vi "LJM_eNames.vi"(0 "Handle In":i32, 1 "NumFrames":i32=-1, 5 "aNames":string[](array[string]), 9 "aValuesIn":dbl[](array[numeric]) format="%.2f", 11 "error in":errorcluster, 12 "aWrites":i32[](array[ring]) items=["Read", "Write"], 13 "aNumValues":i32[](array[numeric])) -> (4 "Handle Out":i32, 10 "aValuesOut":dbl[](array[numeric]) format="%.2f", 14 "ErrorAddress":i32, 15 "error out":errorcluster)   [LabVIEW 2020]
panel:
  # "This function does not check or modify the aValuesIn array.  You must initialize it properly.  We recommend\nalways using eNames2D in LabVIEW rather than eNames."
  # "1/20/2015:  Default value of NumFrames changed to -1.  If\nNumFrames = -1, then the NumFrames control is ignored\nand the size of aNames/aAddresses is used to determine how\nmany frames there are."
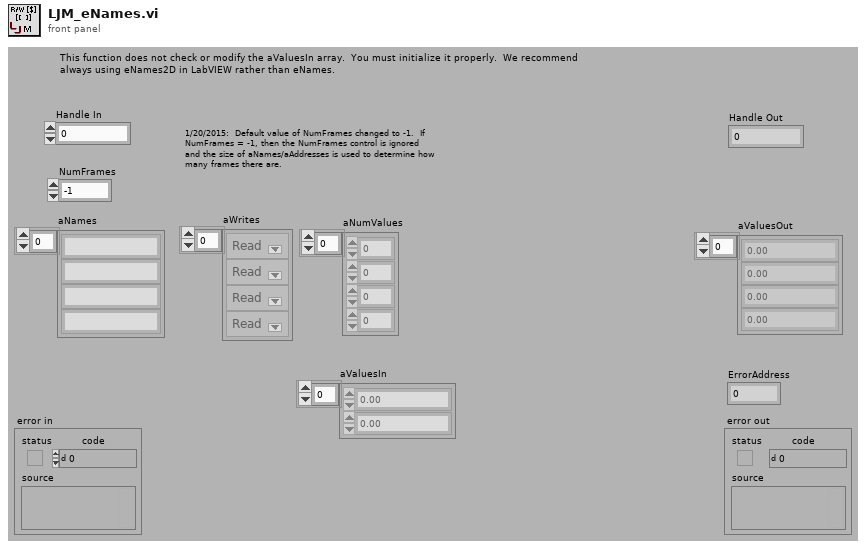
[diagram p1: front panel]
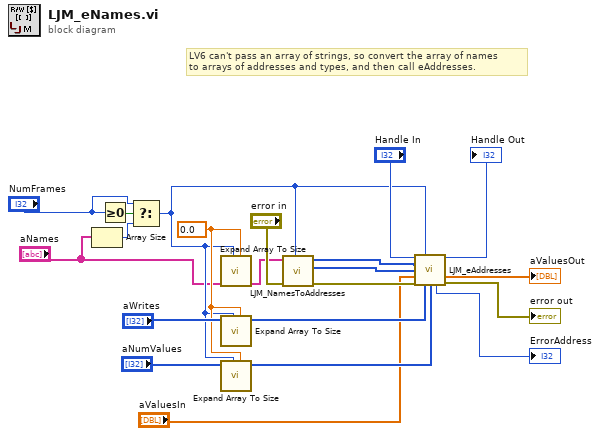
[diagram p0: block diagram]
diagram:
  w7 = 0.0 ("Default Value")
  # "LV6 can't pass an array of strings, so convert the array of names\nto arrays of addresses and types, and then call eAddresses."
  n1 = Array Size(array="aNames") -> (size(s)=w5:i32)
  n2 = Greater Or Equal To 0?(x="NumFrames") -> (x >= 0?=w4:bool)
  n3 = Select(t="NumFrames", s=w4, f=w5) -> (s? t:f=w3:i32)
  n4 = call "Expand Array To Size.vi"("Default Value"=w7, "# Elements"=w3, "String Array In"="aNames") -> ("String Array Out"=w18:string[])  [unwired: 4 in, 4 out]
  n5 = call "Expand Array To Size.vi"("Default Value"=w7, "# Elements"=w3, "I32 Array In"="aWrites") -> ("I32 Array Out"=w12:i32[])  [unwired: 4 in, 4 out]
  n6 = call "Expand Array To Size.vi"("Default Value"=w7, "# Elements"=w3, "I32 Array In"="aNumValues") -> ("I32 Array Out"=w11:i32[])  [unwired: 4 in, 4 out]
  n7 = call "LJM_NamesToAddresses.vi"("NumFrames (Auto-Detect)"=w3, "error in"="error in", "aNames"=w18) -> ("error out"=w17:errorcluster, "aTypes"=w13:i32[], "aAddresses"=w14:i32[])  [unwired: 6 in]
  n8 = call "LJM_eAddresses.vi"("Handle In"="Handle In", "NumFrames"=w3, "aAddresses"=w14, "aTypes"=w13, "aValuesIn"="aValuesIn", "error in"=w17, "aWrites"=w12, "aNumValues"=w11) -> ("Handle Out"=→"Handle Out":i32, "aValuesOut"=→"aValuesOut":dbl[], "ErrorAddress"=→"ErrorAddress":i32, "error out"=→"error out":errorcluster)  [unwired: 4 in]
